vi "Get Wire Type.vi"(8 "error in (no error)":errorcluster, 11 "Wire Type Group in":refnum<class "Wire Type Group.lvclass">) -> (0 "error out":errorcluster, 2 "Wire Type":T1, 3 "Wire Type Group out":refnum<class "Wire Type Group.lvclass">)   [LabVIEW 2020, in "Protobuf RAW.lvlib" / "Wire Type Group.lvclass"]
uses:
  Wire Type Group.lvclass
  Type Serializer/Wire Type.ctl
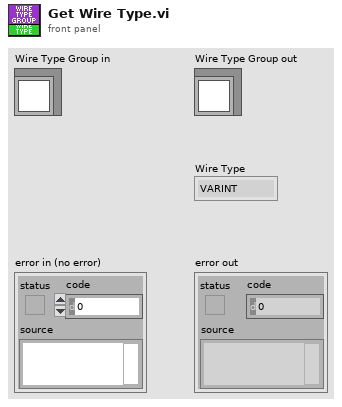
[diagram p1: front panel]
types:
  T1 = typedef "Protobuf RAW.lvlib/Wire Type Group.lvclass/Wire Type.ctl" = enum16{"VARINT", "I64", "LEN", "SGROUP", "EGROUP", "I32"}
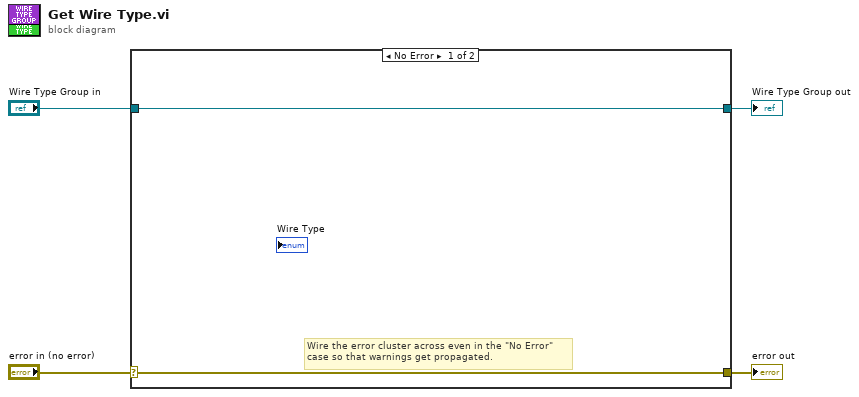
[diagram p0: block diagram]
diagram:
  n1 = case shown="No Error" "error in (no error)" {
    selector: "error in (no error)" -> [w5 w8]
    tunnel: [w5 w8] -> w3
    tunnel: [w6 w7] -> w1
    tunnel: "Wire Type Group in" -> [w6 w7]
    frame No Error {
      # "Wire the error cluster across even in the \"No Error\"\ncase so that warnings get propagated."
    }
    frame Error {
    }
  }
  "error out" <- w3
  "Wire Type Group out" <- w1
